vi "ze advanced subscriber last sample miss detection options default.vi"(8 "error in (no error)":errorcluster, 11 "this_":cluster{}) -> (0 "error out":errorcluster, 3 "this_ out":cluster{})   [LabVIEW 2021, in "zenohc.lvlib"]
doc: "void ze_advanced_subscriber_last_sample_miss_detection_options_default(struct ze_advanced_subscriber_last_sample_miss_detection_options_t *this_);"
uses:
  zenohc.lvlib
  zenohc.dll
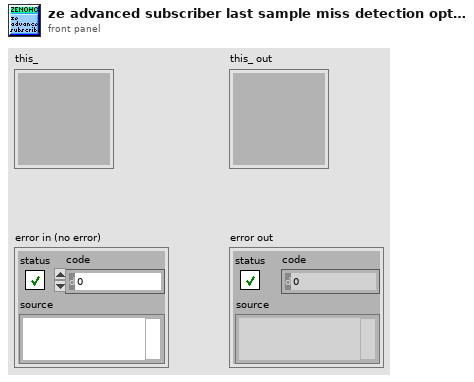
[diagram p1: front panel]
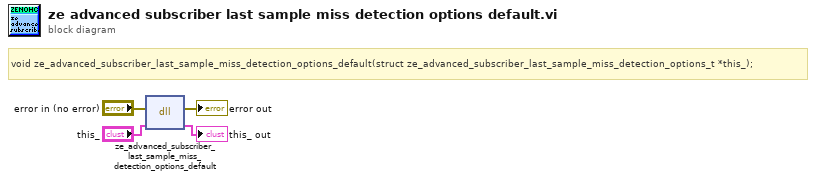
[diagram p0: block diagram]
diagram:
  # "void ze_advanced_subscriber_last_sample_miss_detection_options_default(struct ze_advanced_subscriber_last_sample_miss_detection_options_t *this_);"
  n1 = dll-call lib="D:/dev/zenoh_labview/zenohc/zenohc.*" fn="ze_advanced_subscriber_last_sample_miss_detection_options_default"(error in="error in (no error)", "this_"="this_") -> (error out=→"error out":errorcluster, "this_"=→"this_ out":cluster{})  [unwired: 3 in, 1 out]
